vi "MQTT Send.vi"(8 "error in (no error)":errorcluster, 9 "Payload Full":string, 10 "Topic Name":string, 11 "Client in":refnum<class "Client.lvclass">) -> (0 "error out":errorcluster, 2 "Published":bool, 3 "Client out":refnum<class "Client.lvclass">)   [LabVIEW 2021]
uses:
  <vilib>/LabVIEW Open Source Project/MQTT Client/Client class/Client.lvclass
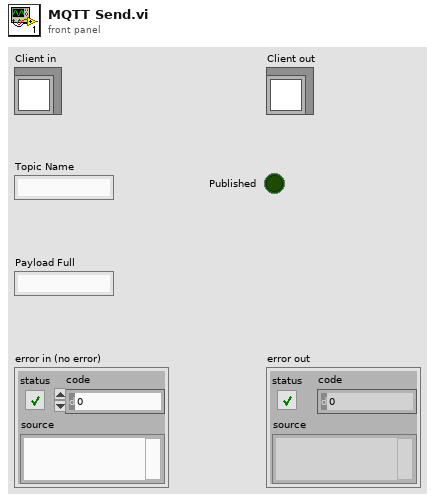
[diagram p1: front panel]
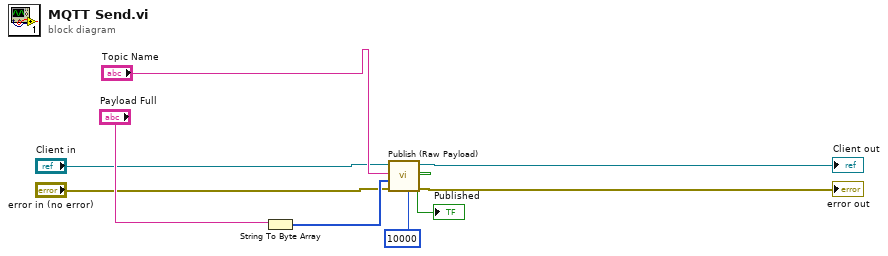
[diagram p0: block diagram]
diagram:
  n1 = String To Byte Array(string="Payload Full") -> (unsigned byte array=w6:u8[])
  n2 = call <vilib>:"Publish (Raw Payload).vi"("timeout (1000ms)"=10000, "error in (no error)"="error in (no error)", "Binary Payload"=w6, "Topic Name"="Topic Name", "Client in"="Client in") -> ("error out"=→"error out":errorcluster, "Published"=→"Published":bool, "Client out"=→"Client out":refnum<class "Client.lvclass">)  [unwired: 4 in]
